vi "DAY 10 EXP1.vi"() -> ()   [LabVIEW 2018]
uses:
  <vilib>/DAQmx/read.llb/DAQmx Read (Analog 1D DBL NChan 1Samp).vi
  <vilib>/DAQmx/write.llb/DAQmx Write (Analog DBL 1Chan 1Samp).vi
  <vilib>/Analysis/1siggen.llb/Ramp Pattern by Delta.vi
  <vilib>/DAQmx/create/channels.llb/DAQmx Create Channel (AO-Voltage-Basic).vi
  <vilib>/DAQmx/create/channels.llb/DAQmx Create Channel (AI-Voltage-Basic).vi
  <vilib>/DAQmx/miscellaneous.llb/DAQmx Fill In Error Info.vi
  <vilib>/Analysis/NI_AALBase.lvlib
panel:
  out "XY Graph":cluster{dbl[], dbl[]}(graph)
  in  "physical channels 2":tag
  in  "physical channels":tag
  in  "delta":dbl=0.2 format="%#_13g"
  out "Ramp Pattern":dbl[](array[numeric])
  in  "start":dbl
  in  "end":dbl=1.0
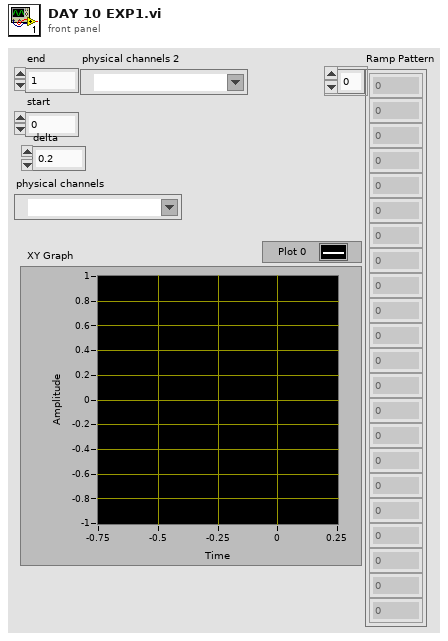
[diagram p1: front panel]
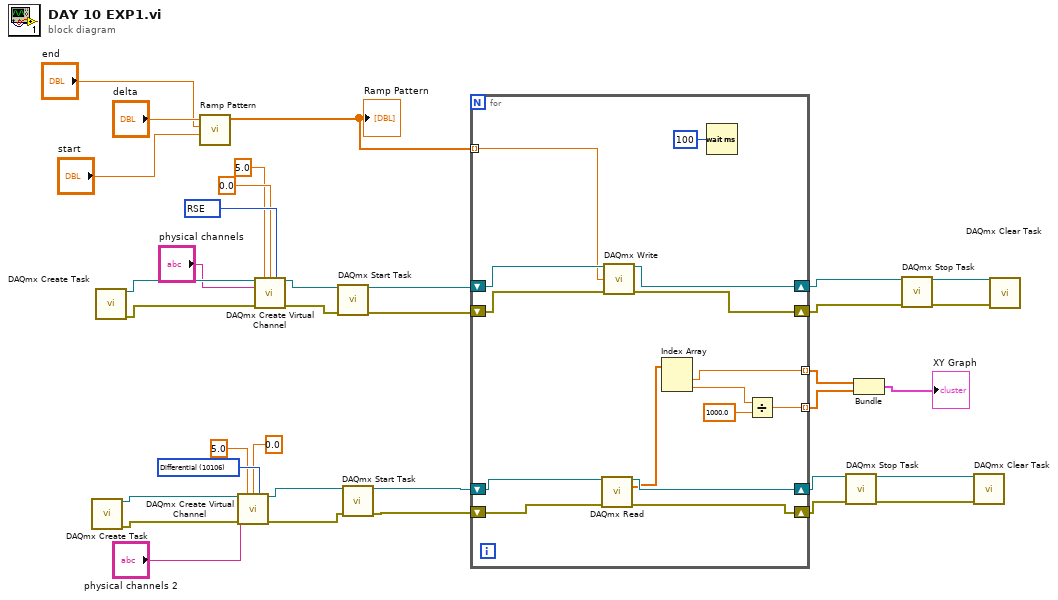
[diagram p0: block diagram]
diagram:
  w11 = 10106 items=["Default"=-1, "RSE"=10083, "NRSE"=10078, "Differential"=10106, "Pseudodifferential"=12529] ("input terminal configuration")
  w31 = 10083 items=["Default"=-1, "RSE"=10083, "Differential"=10106, "Pseudodifferential"=12529] ("output terminal configuration")
  n1 = call <vilib>:"DAQmx Create Task.vi"() -> ("task out"=w8:refnum<k21>, "error out"=w7:errorcluster)  [unwired: 14 in]
  n2 = call <vilib>:"DAQmx Create Task.vi"() -> ("task out"=w18:refnum<k21>, "error out"=w17:errorcluster)  [unwired: 14 in]
  n3 = call-poly <vilib>:"Ramp Pattern.vi"("start"="start", "end"="end", "delta"="delta") -> ("Ramp Pattern"=w32:dbl[])  [unwired: 6 in, 2 out]
  "Ramp Pattern" <- w32
  n4 = call-poly <vilib>:"DAQmx Create Virtual Channel.vi"("task in"=w8, "maximum value"=5.0, "minimum value"=0.0, "input terminal configuration"=w11, "physical channels"="physical channels 2", "error in"=w7) -> ("task out"=w5:refnum<k21>, "error out"=w4:errorcluster)  [unwired: 8 in]
  n5 = call-poly <vilib>:"DAQmx Create Virtual Channel.vi"("task in"=w18, "maximum value"=5.0, "minimum value"=0.0, "output terminal configuration"=w31, "physical channels"="physical channels", "error in"=w17) -> ("task out"=w15:refnum<k21>, "error out"=w14:errorcluster)  [unwired: 8 in]
  n6 = call <vilib>:"DAQmx Start Task.vi"("task/channels in"=w15, "error in"=w14) -> ("task out"=w26:refnum<k21>, "error out"=w25:errorcluster)  [unwired: 12 in]
  n7 = call <vilib>:"DAQmx Start Task.vi"("task/channels in"=w5, "error in"=w4) -> ("task out"=w13:refnum<k21>, "error out"=w12:errorcluster)  [unwired: 12 in]
  n8 = for {
    tunnel: w32 -> [w44] mode=indexing
    shift-right: [w50] -> w28
    shift-left: w26 -> [w48]
    shift-right: [w49] -> w27
    shift-left: w25 -> [w47]
    shift-right: [w46] -> w22
    shift-left: w13 -> [w42]
    shift-right: [w45] -> w20
    shift-left: w12 -> [w43]
    tunnel: [w40] -> w2 mode=indexing
    tunnel: [w39] -> w3 mode=indexing
    n9 = call-poly <vilib>:"DAQmx Read.vi"("task/channels in"=w42, "error in"=w43) -> ("task out"=w46:refnum<k21>, "data"=w38:dbl[], "error out"=w45:errorcluster)  [unwired: 11 in]
    n10 = call-poly <vilib>:"DAQmx Write.vi"("task/channels in"=w48, "data"=w44, "error in"=w47) -> ("task out"=w50:refnum<k21>, "error out"=w49:errorcluster)  [unwired: 10 in, 1 out]
    n11 = Index Array(array=w38) -> (element #1=w39:dbl, element #2=w37:dbl)  [unwired: 2 in]
    n12 = Wait (ms)(milliseconds to wait=u32 100) -> ()  [unwired: 1 out]
    n13 = Divide(x=w37, y=1000.0) -> (x/y=w40:dbl)
  }
  n14 = call <vilib>:"DAQmx Stop Task.vi"("task/channels in"=w22, "error in"=w20) -> ("task out"=w21:refnum<k21>, "error out"=w19:errorcluster)  [unwired: 12 in]
  n15 = Bundle(w3, w2) -> (→"XY Graph":cluster{dbl[], dbl[]})  [unwired: 1 in]
  n16 = call <vilib>:"DAQmx Stop Task.vi"("task/channels in"=w28, "error in"=w27) -> ("task out"=w24:refnum<k21>, "error out"=w23:errorcluster)  [unwired: 12 in]
  n17 = call <vilib>:"DAQmx Clear Task.vi"("task in"=w21, "error in"=w19) -> ()  [unwired: 13 in, 1 out]
  n18 = call <vilib>:"DAQmx Clear Task.vi"("task in"=w24, "error in"=w23) -> ()  [unwired: 13 in, 1 out]
